vi "波形存储(子VI).vi"(11 "ORP滴定曲线":u16[](graph)) -> ()   [LabVIEW 2016, in "斯坦道CODMn.lvlib"]
uses:
  <vilib>/Utility/sysdir.llb/System Directory Type.ctl
  <vilib>/Waveform/WDTFileIO.llb/ Write Waveform to File.vi
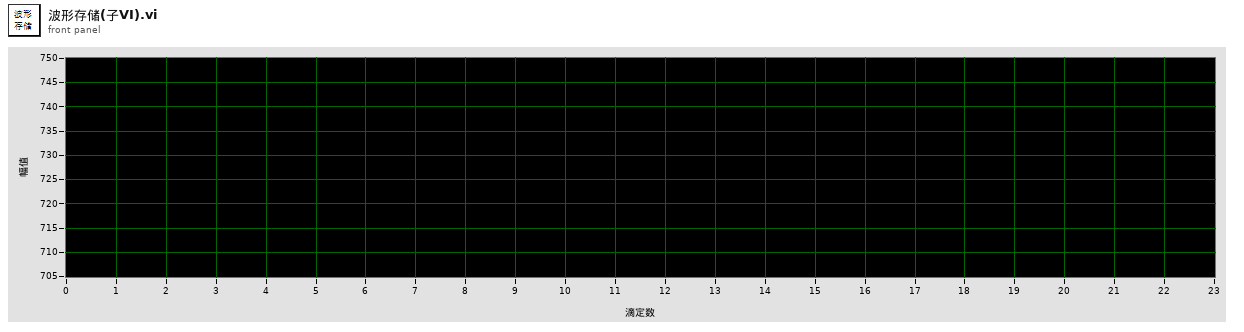
[diagram p1: front panel]
types:
  T1 = typedef "System Directory Type.ctl" = i32
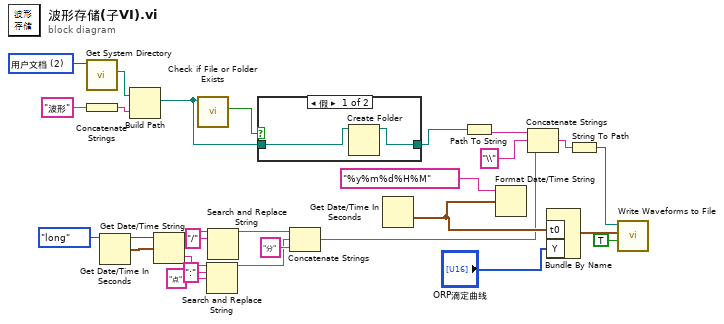
[diagram p0: block diagram]
diagram:
  w15 = T1 2 items=["用户目录"=0, "用户桌面"=1, "用户文档"=2, "用户应用程序数据"=3, "用户设置"=4, "用户临时目录"=5, "公共文档"=6, "公共应用程序数据"=7, "公共设置"=8, "公共缓存"=13, "系统核心库"=9, "系统安装库"=10, "应用程序文件"=11, "启动盘根目录"=12] ("system directory type")
  n1 = call <vilib>:"Get System Directory.vi"("system directory type"=w15) -> ("system directory"=w14:path)  [unwired: 10 in]
  n2 = Concatenate Strings("波形" ("condition")) -> (w12:string)
  n3 = Get Date/Time In Seconds() -> (seconds since 1Jan1904=w2:timestamp)
  n4 = Build Path(base path=w14, name or relative path=w12) -> (appended path=w17:path)
  n5 = Get Date/Time String(date format (0)=enum16{"short", "long", "abbreviated"}."long" ("日期格式(0)"), seconds (now)=w2) -> (date string=w5:string, time string=w7:string)  [unwired: 1 in]
  n6 = call <vilib>:"Check if File or Folder Exists.vi"("path"=w17) -> ("file or folder exists?"=w16:bool)  [unwired: 8 in, 2 out]
  n7 = Search and Replace String(input string=w7, search string=":" ("搜索字符串"), replace string="点" ("替换字符串(\"\")")) -> (result string=w9:string)  [unwired: 5 in, 3 out]
  n8 = Search and Replace String(input string=w5, search string="/" ("搜索字符串")) -> (result string=w4:string)  [unwired: 6 in, 3 out]
  n9 = case shown="假" w16 {
    tunnel: w17 -> [w29 w30]
    tunnel: [w28 w30] -> w26
    frame False {
      n10 = Create Folder(path (use dialog)=w29) -> (created path=w28:path)  [unwired: 2 in, 2 out]
    }
    frame True {
    }
  }
  n11 = Concatenate Strings(w4, w9, "分" ("字符串")) -> (w1:string)
  n12 = Get Date/Time In Seconds() -> (seconds since 1Jan1904=w23:timestamp)
  n13 = Path To String(path=w26) -> (string=w19:string)
  n14 = Format Date/Time String(time format string (%c)="%y%m%d%H%M" ("时间格式字符串(%c)"), seconds (now)=w23) -> ()  [unwired: 1 in, 1 out]
  n15 = Concatenate Strings(w19, "\\" ("字符串"), w1) -> (w21:string)
  n16 = Bundle By Name("t0"=w23, "Y"="ORP滴定曲线") -> (w18:waveform(u16))  [unwired: 1 in]
  n17 = String To Path(string=w21) -> (path=w22:path)
  n18 = call-poly <vilib>:"Write Waveforms to File.vi"("append to file? (new file:F)"=TRUE, "waveform"=w18, "file path (dialog if empty)"=w22) -> ()  [unwired: 7 in, 2 out]
